vi "Switch Sides.vi"(10 "Side":enum16{"Esquerdo", "Direito"}(ring) caption="Enum", 11 "Camera State Input.lvclass":refnum<class "Camera.lvclass">) -> (3 "Camera State Side Mirrored.lvclass":refnum<class "Camera.lvclass">)   [LabVIEW 2018]
uses:
  Camera_class/Camera.lvclass
  Camera_class/Camera.lvclass/Camera.ctl
  Object_class/Object.lvclass/Object.ctl
  Robot_class/Robot.lvclass/Robot.ctl
  Object_class/Read x.vi
  Object_class/Read y.vi
  Object_class/Write x.vi
  Object_class/Write y.vi
  <vilib>/Analysis/coordinate.llb/Wrap Angle (scalar).vi
  Robot_class/Read orientation.vi
  Robot_class/Write orientation.vi
  Camera_class/Read Balls.vi
  Camera_class/Write Balls.vi
  Ball_class/Ball.lvclass
  C:/Users/Ronaldo/Desktop/Phoenix/SSL_AI/Object_class/Object.lvclass
  Robot_class/Robot.lvclass
  <vilib>/Analysis/NI_AAL_Angle.lvlib
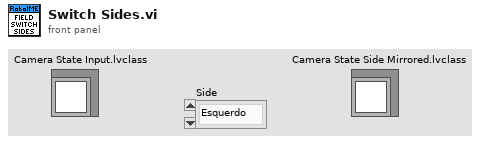
[diagram p1: front panel]
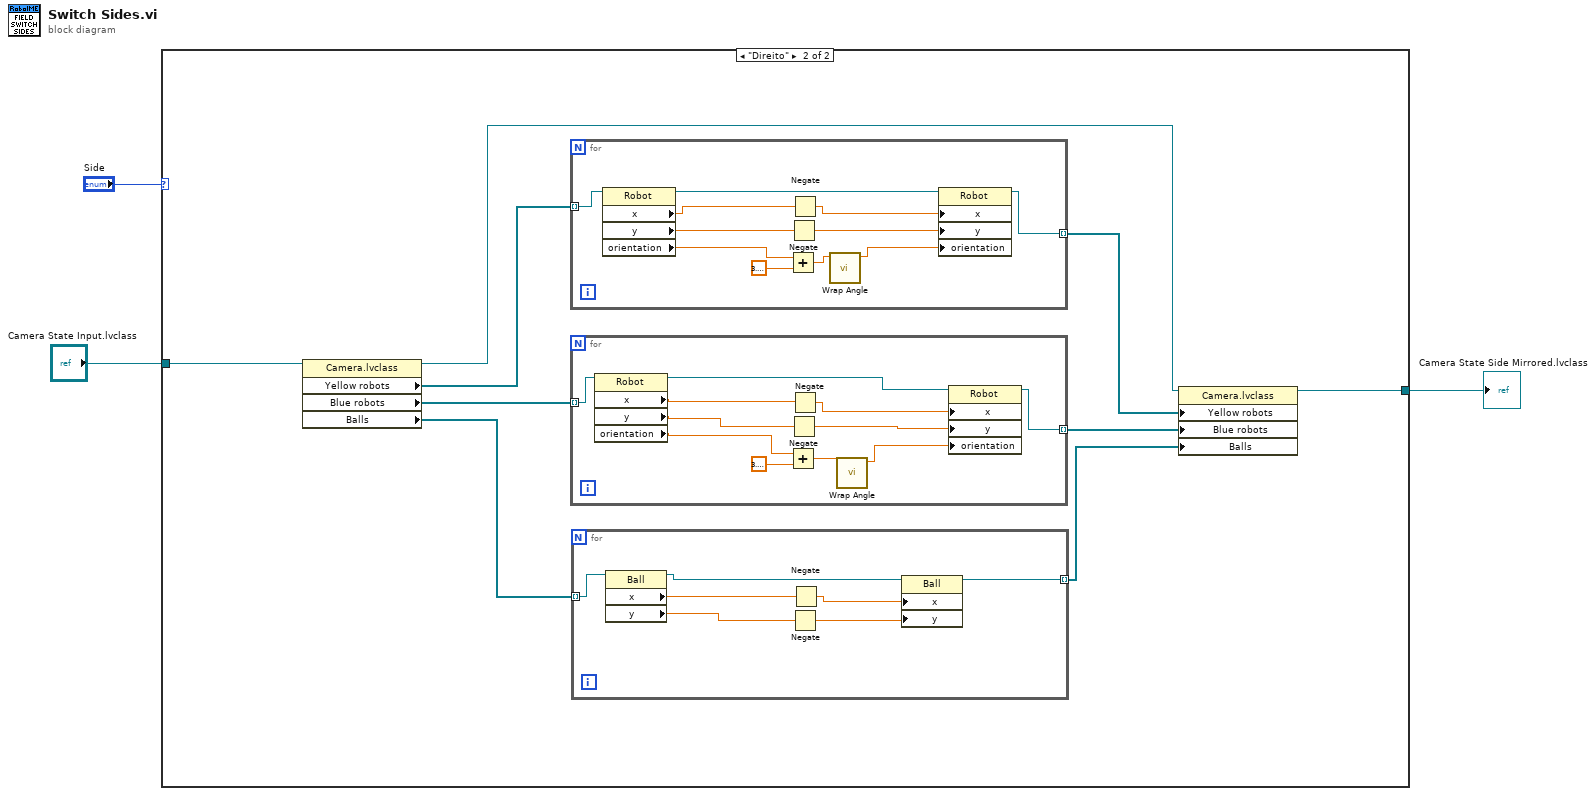
[diagram p0: block diagram]
diagram:
  n1 = case shown="\"Direito\"" "Side" {
    tunnel: [w4 w7] -> w3
    tunnel: "Camera State Input.lvclass" -> [w4 w6]
    frame "Esquerdo", Default {
    }
    frame "Direito" {
      n2 = property class="Camera.lvclass"(reference=w6) -> (reference out=w5:refnum<class "Camera.lvclass">, "Yellow robots"=w13:refnum<class "Robot.lvclass">[], "Blue robots"=w12:refnum<class "Robot.lvclass">[], "Balls"=w11:refnum<class "Ball.lvclass">[])  [unwired: 1 in, 1 out]
      n3 = for {
        tunnel: w13 -> [w40] mode=indexing
        tunnel: [w32] -> w10 mode=indexing
        n4 = property class="Robot"(reference=w40) -> (reference out=w36:refnum<class "Robot.lvclass">, "x"=w39:dbl, "y"=w38:dbl, "orientation"=w37:dbl)  [unwired: 1 in, 1 out]
        n5 = Add(x=w37, y=3.141592653589793) -> (x+y=w41:dbl)
        n6 = Negate(x=w38) -> (-x=w34:dbl)
        n7 = Negate(x=w39) -> (-x=w35:dbl)
        n8 = call-poly <vilib>:"Wrap Angle.vi"("angle in"=w41) -> ("angle out"=w33:dbl)  [unwired: 9 in, 1 out]
        n9 = property class="Robot"(reference=w36, "x"=w35, "y"=w34, "orientation"=w33) -> (reference out=w32:refnum<class "Robot.lvclass">)  [unwired: 1 in, 1 out]
      }
      n10 = for {
        tunnel: w12 -> [w19] mode=indexing
        tunnel: [w15] -> w9 mode=indexing
        n11 = property class="Robot"(reference=w19) -> (reference out=w14:refnum<class "Robot.lvclass">, "x"=w20:dbl, "y"=w21:dbl, "orientation"=w22:dbl)  [unwired: 1 in, 1 out]
        n12 = Add(x=w22, y=3.141592653589793) -> (x+y=w23:dbl)
        n13 = Negate(x=w21) -> (-x=w17:dbl)
        n14 = Negate(x=w20) -> (-x=w18:dbl)
        n15 = call-poly <vilib>:"Wrap Angle.vi"("angle in"=w23) -> ("angle out"=w16:dbl)  [unwired: 9 in, 1 out]
        n16 = property class="Robot"(reference=w14, "x"=w18, "y"=w17, "orientation"=w16) -> (reference out=w15:refnum<class "Robot.lvclass">)  [unwired: 1 in, 1 out]
      }
      n17 = for {
        tunnel: w11 -> [w31] mode=indexing
        tunnel: [w26] -> w8 mode=indexing
        n18 = property class="Ball"(reference=w31) -> (reference out=w25:refnum<class "Ball.lvclass">, "x"=w30:dbl, "y"=w29:dbl)  [unwired: 1 in, 1 out]
        n19 = Negate(x=w29) -> (-x=w27:dbl)
        n20 = Negate(x=w30) -> (-x=w28:dbl)
        n21 = property class="Ball"(reference=w25, "x"=w28, "y"=w27) -> (reference out=w26:refnum<class "Ball.lvclass">)  [unwired: 1 in, 1 out]
      }
      n22 = property class="Camera.lvclass"(reference=w5, "Yellow robots"=w10, "Blue robots"=w9, "Balls"=w8) -> (reference out=w7:refnum<class "Camera.lvclass">)  [unwired: 1 in, 1 out]
    }
  }
  "Camera State Side Mirrored.lvclass" <- w3
